vi "TalkTracker_group.vi"(0 "PORT NAME":string="Inlet_Heaters", 1 "Set":enum16{"Set", "Read"}(ring), 3 "Value to set":dbl, 9 "LOCATION":i32=15, 11 "NO. LOCATIONS":i32=1, 12 "Analogue":enum16{"Logic", "Analogue"}(ring)) -> ()   [LabVIEW 2010]
panel:
  out "Comments":string[](array[string])
  out "Responses":string[](array[string])
  in  "Module Addresses":i32[](array[numeric])=[101, 102, 103, 104, 105, 106, 107, 108, 109, 110, 111, 112, 113, 114, 115]
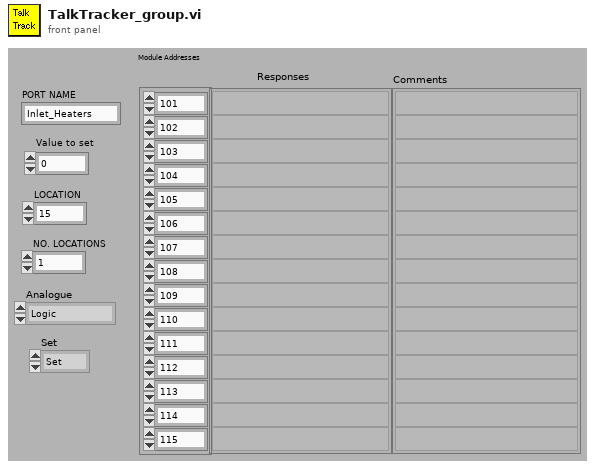
[diagram p1: front panel]
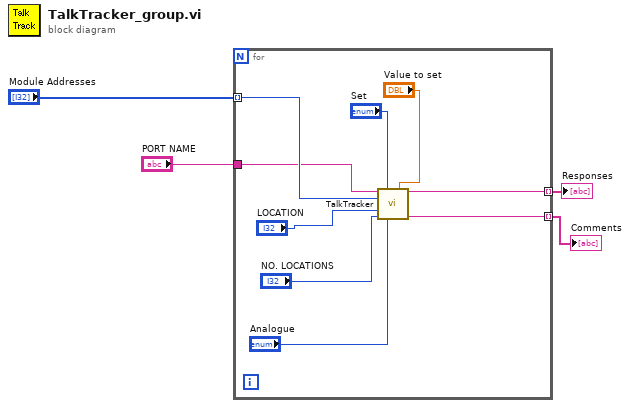
[diagram p0: block diagram]
diagram:
  n1 = for {
    tunnel: "Module Addresses" -> [w13] mode=indexing
    tunnel: [w7] -> w3 mode=indexing
    tunnel: [w6] -> w1 mode=indexing
    tunnel: "PORT NAME" -> [w5]
    n2 = call "TalkTracker.vi"("PORT NAME"=w5, "Set"="Set", "Value to set"="Value to set", "MODULE ADDRESS"=w13, "LOCATION"="LOCATION", "NO. LOCATIONS"="NO. LOCATIONS", "Analogue"="Analogue") -> ("Response"=w7:string, "Comment out"=w6:string)  [unwired: 6 in, 1 out]
  }
  "Responses" <- w3
  "Comments" <- w1
